vi "Drivetrain Loop.vi"() -> ()   [LabVIEW 2015]
uses:
  Common Code/Drivetrain Modes.ctl
  Common Code/Change Detect Boolean.vi
  Robot Global Data.vi
  <vilib>/Rock Robotics/WPI/Solenoid/Deprecated/WPI_SolenoidSetBool.vi
panel:
  out "Modes":T1=enum."Goal Vision Targeting"
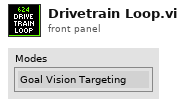
[diagram p1: front panel]
types:
  T1 = typedef "Drivetrain Modes.ctl" = enum16{"Gyro Steer", "Climb", "Manual", "Goal Vision Targeting", "PID Distance Drive", "Hybrid"}
  T2 = typedef "Drivetrain Commands.ctl" = cluster{"Y Power":dbl, "Turn Power":dbl, "Modes":T1, "Heading Target":dbl, "X Max Speed":dbl, "Y Max Speed":dbl, "X Min Speed":dbl, "Y Min Speed":dbl, "Y Target":dbl, "Max Accel":dbl, "Max Velocity":dbl, "Pivot Speed":dbl}
  T3 = typedef "WPI_DriverStationRobotMode2.ctl" = enum16{"Autonomous Disabled", "Autonomous Enabled", "Teleop Disabled", "Teleop Enabled", "Disconnected", "Finish", "Test Disabled", "Test Enabled", "Emergency Stopped"}
  T4 = typedef "Goal Vision Packet.ctl" = cluster{"Distance":dbl, "Center X":dbl, "Center Y":dbl, "Found Target?":bool, "Robot Center":dbl, "Angle":dbl}
  T5 = typedef "Dist Drive Status.ctl" = cluster{"Y In Range":bool, "X In Range":bool, "Gyro In Range":bool, "Y Dist":dbl, "X Dist":dbl, "Gyro":dbl}
  T6 = typedef "WPI_MotorControlDeviceRef.ctl" = cluster{"DeviceStatus":errorcluster, "Type":T7, "PWM":cluster{"PWM Channel":T8, "DeadBand":T9}, "CAN":cluster{"Device Number":u8, "Control Mode":T10, "Semaphore":T11, "Max Vout":dbl, "TalonSRX Control Mode":T12}, "Invert":bool}
  T7 = typedef "WPI_MotorControlType.ctl" = enum16{"PWM", "CAN", "CANTalonSRX"}
  T8 = typedef "FPGA_DIOPWMChannel.ctl" = enum8{"PWM 0", "PWM 1", "PWM 2", "PWM 3", "PWM 4", "PWM 5", "PWM 6", "PWM 7", "PWM 8", "PWM 9", "PWM MXP 0", "PWM MXP 1", "PWM MXP 2", "PWM MXP 3", "PWM MXP 4", "PWM MXP 5", "PWM MXP 6", "PWM MXP 7", "PWM MXP 8", "PWM MXP 9", "Invalid"}
  T9 = typedef "WPI_PWMDeadband.ctl" = cluster{"Name":string, "maxPositivePwm":i32, "minPositivePwm":i32, "centerPwm":i32, "maxNegativePwm":i32, "minNegativePwm":i32, "angularRange":u16}
  T10 = typedef "WPI_CANJaguar_ControlMode.ctl" = enum8{"Percent VBus", "Current", "Speed", "Position", "Voltage"}
  T11 = typedef "Semaphore RefNum" = refnum<k1>
  T12 = typedef "WPI_CANTalonSRX_APIControlMode.ctl" = enum8{"Percent VBus", "Speed", "Position", "Slave", "Unchanged / Invalid", "Voltage Compensation", "Current", "Motion Profile"}
  T13 = typedef "WPI_SolenoidDevRef.ctl" = cluster{"DevStatus":errorcluster, "Pneumatics Control Module":u8, "Forward Solenoid Channel":T14, "Reverse Solenoid Channel":T14}
  T14 = typedef "WPI_SolenoidChannel.ctl" = enum8{"Solenoid 0", "Solenoid 1", "Solenoid 2", "Solenoid 3", "Solenoid 4", "Solenoid 5", "Solenoid 6", "Solenoid 7", "Invalid"}
  T15 = typedef "Drivetrain Status Cluster.ctl" = cluster{"Modes":T1, "Y (Throttle)":dbl, "X (Steer)":dbl, "Gyro In Range?":bool, "Distance Drive Finished?":bool, "Stop Eject Lockout":bool, "Dist Drive Status":T5, "Y Target":dbl, "Heading Target":dbl, "Vision Target Aligned?":bool}
  T16 = typedef "Climb Status Cluster.ctl" = cluster{"Pull Power":dbl, "Unpin Power":dbl, "PTO Engaged?":bool, "Climb Mode":T17}
  T17 = typedef "Climb Mode.ctl" = enum16{"Auto", "Semi-Auto", "Manual"}
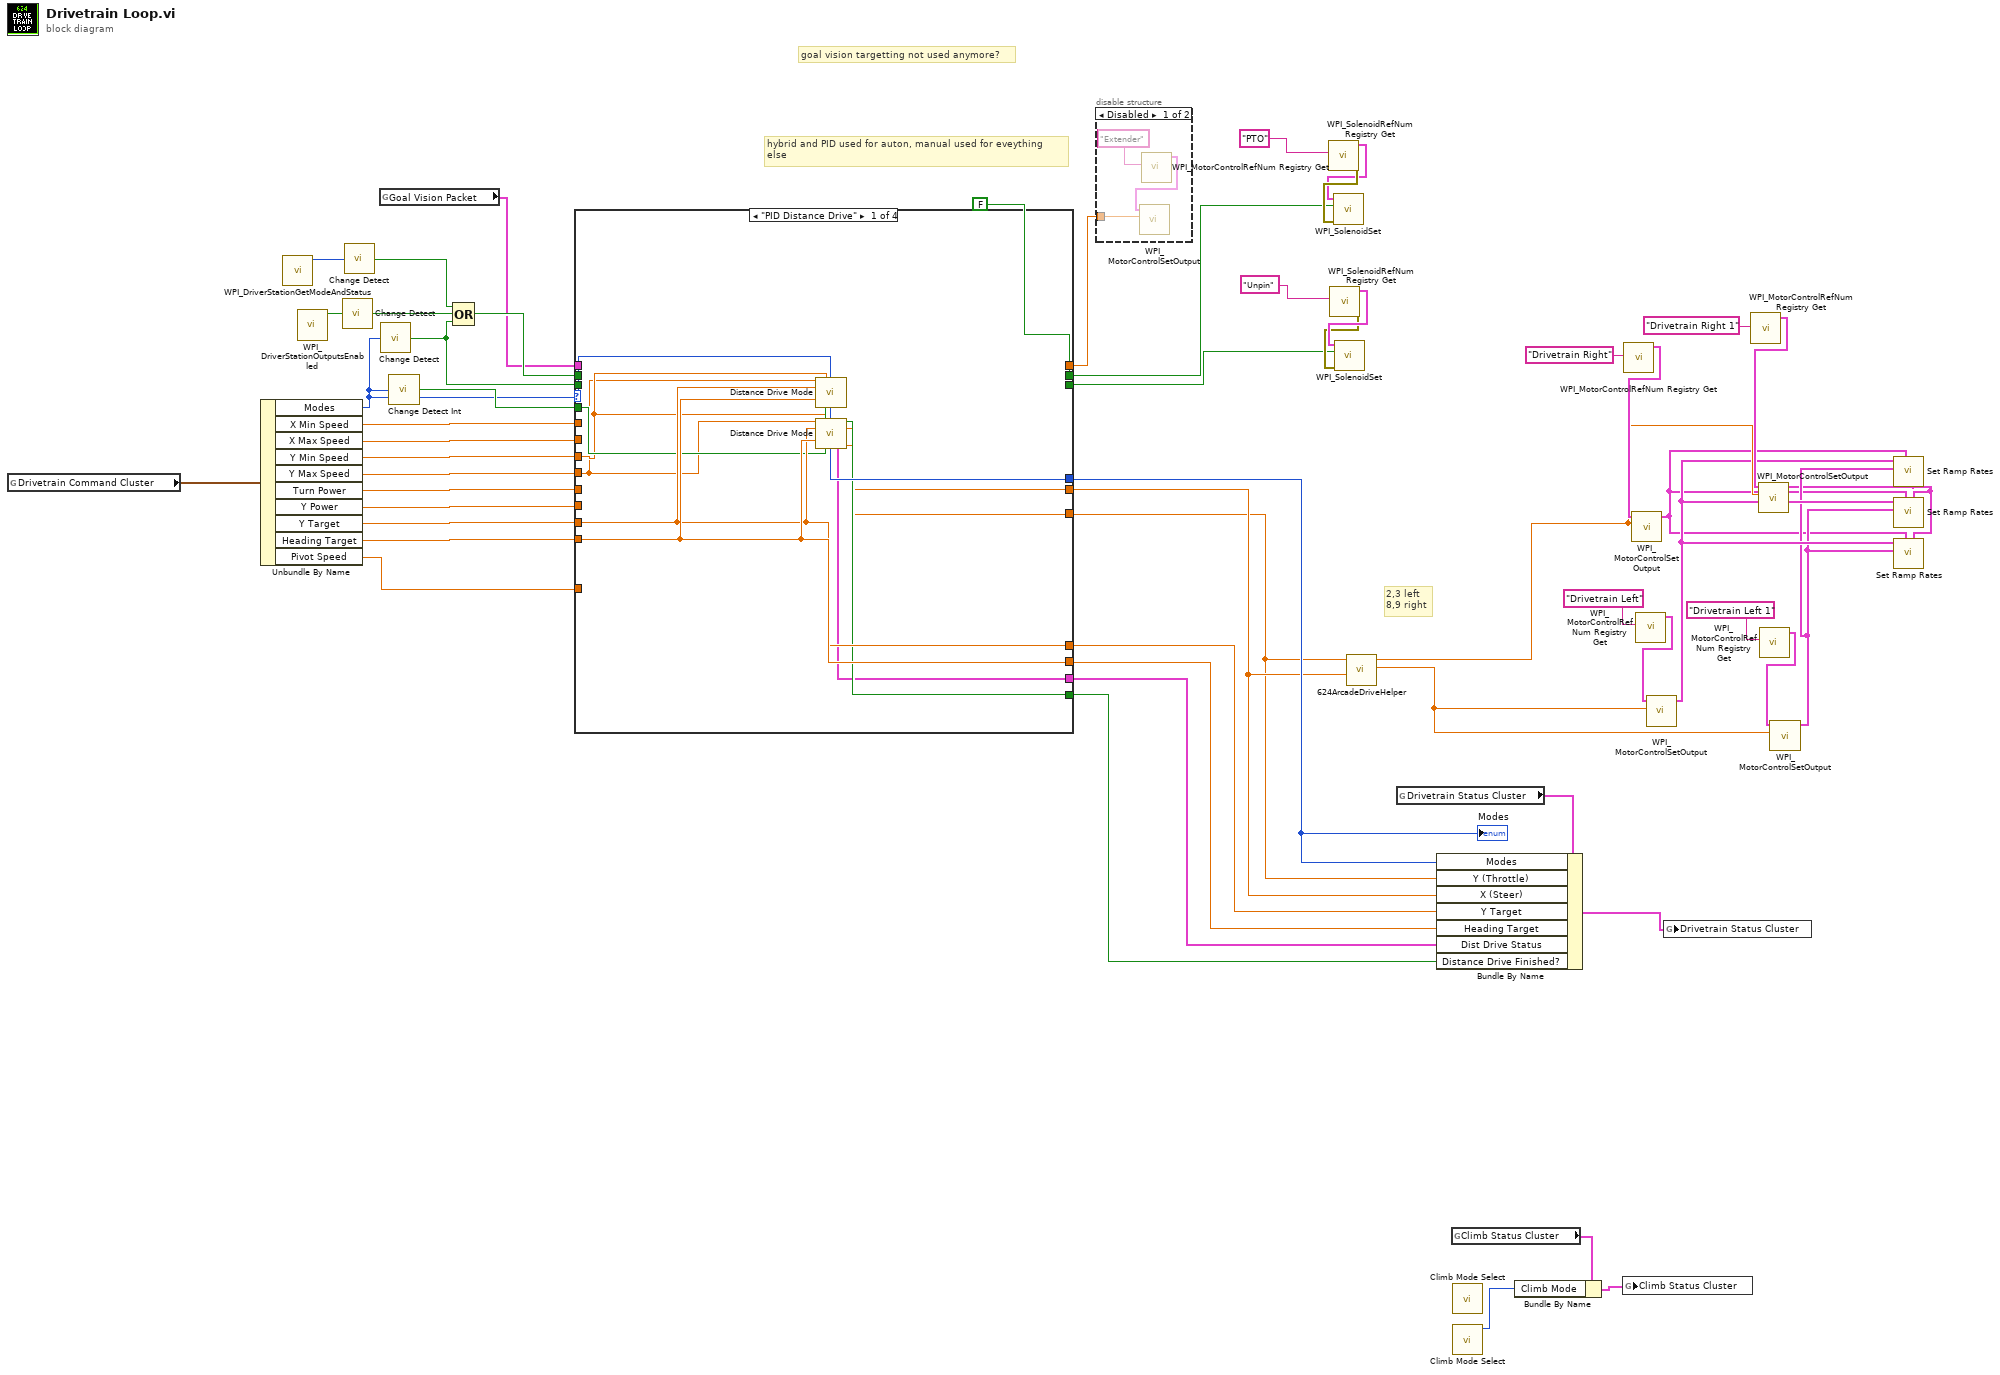
[diagram p0: block diagram]
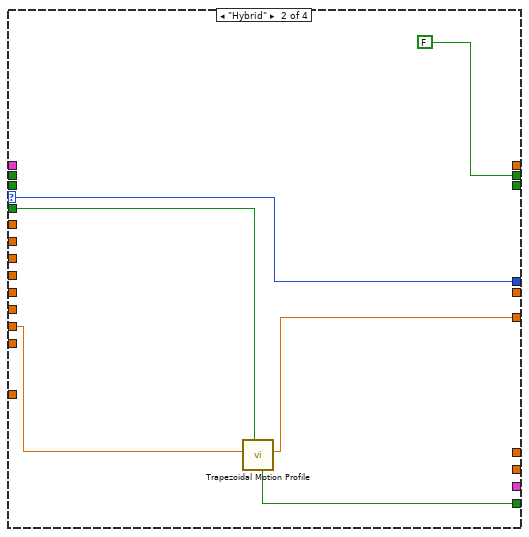
[diagram p3: hidden frame]
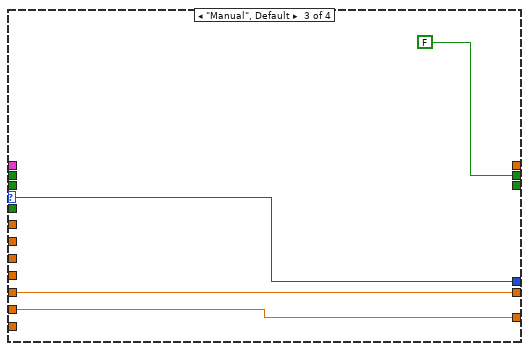
[diagram p4: hidden frame]
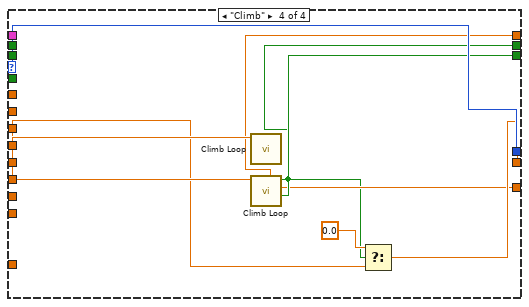
[diagram p5: hidden frame]
diagram:
  # "hybrid and PID used for auton, manual used for eveything \nelse"
  # "goal vision targetting not used anymore?"
  # "2,3 left\n8,9 right"
  n1 = global read "Robot Global Data.vi" "Drivetrain Command Cluster"() -> (w27:T2)
  n2 = Unbundle By Name(w27) -> ("Modes"=w26:T1, "X Min Speed"=w35:dbl, "X Max Speed"=w34:dbl, "Y Min Speed"=w33:dbl, "Y Max Speed"=w32:dbl, "Turn Power"=w31:dbl, "Y Power"=w30:dbl, "Y Target"=w29:dbl, "Heading Target"=w28:dbl, "Pivot Speed"=w2:dbl)
  n3 = call <vilib>:"WPI_DriverStationGetModeAndStatus.vi"() -> ("Robot Mode"=w15:T3)  [unwired: 10 in, 1 out]
  n4 = call <vilib>:"WPI_DriverStationOutputsEnabled.vi"() -> ("OutputsEnabled?"=w17:bool)  [unwired: 10 in, 1 out]
  n5 = call-poly "Change Detect.vi"("In"=w17) -> ("Changed?"=w16:bool)
  n6 = call-poly "Change Detect.vi"("In"=w15) -> ("Changed?"=w14:bool)
  n7 = global read "Robot Global Data.vi" "Goal Vision Packet"() -> (w4:T4)
  n8 = call-poly "Change Detect.vi"("In"=w26) -> ("Changed?"=w13:bool)
  n9 = call "Change Detect Int.vi"("In"=w26) -> ("Changed?"=w51:bool)
  n10 = Compound Arithmetic op=OR(w14, w16, w13) -> (w25:bool)
  n11 = case shown="\"PID Distance Drive\"" w26 {
    selector: w26 -> [w65 w66 w75 w84]
    tunnel: w35 -> [_ _ _ _]
    tunnel: w34 -> [_ _ _ _]
    tunnel: w33 -> [w60 _ _ _]
    tunnel: [w57 w71 w74 w78] -> w3
    tunnel: [w55 _ w72 w82] -> w24
    tunnel: [w65 w66 w75 w84] -> w54
    tunnel: w51 -> [w61 w69 _ _]
    tunnel: [w56 _ _ _] -> w46
    tunnel: [w58 w70 _ _] -> w47
    tunnel: [w63 _ _ _] -> w45
    tunnel: [w64 _ _ _] -> w44
    tunnel: w32 -> [w59 _ _ _]
    tunnel: w31 -> [_ _ w72 w80]
    tunnel: w30 -> [_ _ w74 w83]
    tunnel: w28 -> [w64 _ _ _]
    tunnel: w29 -> [w63 w68 _ _]
    tunnel: w4 -> [_ _ _ _]
    tunnel: [_ _ _ w76] -> w36
    tunnel: [FALSE ("PTO Engage") FALSE ("PTO Engage") FALSE ("PTO Engage") w77] -> w39
    tunnel: w2 -> [_ _ _ _]
    tunnel: w25 -> [_ _ _ _]
    tunnel: w13 -> [_ _ _ _]
    tunnel: [_ _ _ w79] -> w9
    frame "PID Distance Drive" {
      n12 = call "Distance Drive Mode.vi"("Y Output High"=w59, "Y Output Low"=w60, "Y target"=w63, "Heading target"=w64, "Reinitialize"=w61) -> ()  [unwired: 7 in, 4 out]
      n13 = call "Distance Drive Mode.vi"("Y Output High"=w59, "Y Output Low"=w60, "Y target"=w63, "Heading target"=w64, "Reinitialize"=w61) -> ("isFinished"=w58:bool, "Y out"=w57:dbl, "Dist Drive Status"=w56:T5, "X out"=w55:dbl)  [unwired: 7 in]
    }
    frame "Hybrid" {
      n14 = call "Trapezoidal Motion Profile.vi"("Reset?"=w69, "Distance"=w68) -> ("Throttle Out"=w71:sgl, "Finished?"=w70:bool)  [unwired: 8 in]
    }
    frame "Manual", Default {
    }
    frame "Climb" {
      n15 = call "Climb Loop.vi"("Y Power"=w83) -> ()  [unwired: 7 in, 4 out]
      n16 = call "Climb Loop.vi"("Y Power"=w83) -> ("Unpin?"=w79:bool, "Pull Power"=w78:dbl, "PTO Engaged?"=w77:bool, "Extend Power"=w76:dbl)  [unwired: 7 in]
      n17 = Select(t=0.0, s=w77, f=w80) -> (s? t:f=w82:dbl)
    }
  }
  "Modes" <- w54
  n18 = disable-structure shown="Disabled" {
    disable-tunnel: w36 -> [w87 _]
    frame Disabled {
      n19 = call <vilib>:"WPI_MotorControlRefNum Registry Get.vi"("refnum name"="Extender") -> ("MotorControlDevRef"=w86:T6)  [unwired: 9 in, 1 out]
      n20 = call <vilib>:"WPI_MotorControlSetOutput.vi"("Output"=w87, "MotorControlDevRef"=w86) -> ()  [unwired: 7 in, 3 out]
    }
    frame Enabled {
    }
  }
  n21 = call <vilib>:"WPI_SolenoidRefNum Registry Get.vi"("refnum name"="PTO") -> ("error out"=w42:errorcluster, "SolenoidDevRef"=w41:T13)  [unwired: 9 in]
  n22 = call <vilib>:"WPI_SolenoidRefNum Registry Get.vi"("refnum name"="Unpin") -> ("error out"=w10:errorcluster, "SolenoidDevRef"=w11:T13)  [unwired: 9 in]
  n23 = call-poly <vilib>:"WPI_SolenoidSet.vi"("error in (no error)"=w42, "Value"=w39, "SolenoidDevRef"=w41) -> ()  [unwired: 7 in, 2 out]
  n24 = call-poly <vilib>:"WPI_SolenoidSet.vi"("error in (no error)"=w10, "Value"=w9, "SolenoidDevRef"=w11) -> ()  [unwired: 7 in, 2 out]
  n25 = call "624ArcadeDriveHelper.vi"("Turn Power"=w24, "Y Power"=w3) -> ("Left"=w21:dbl, "Right"=w18:dbl)  [unwired: 8 in]
  n26 = global read "Robot Global Data.vi" "Drivetrain Status Cluster"() -> (w43:T15)
  n27 = Bundle By Name(cluster=w43, "Modes"=w54, "Y (Throttle)"=w3, "X (Steer)"=w24, "Y Target"=w45, "Heading Target"=w44, "Dist Drive Status"=w46, "Distance Drive Finished?"=w47) -> (w48:T15)
  n28 = global read "Robot Global Data.vi" "Climb Status Cluster"() -> (w37:T16)
  n29 = call "Climb Mode Select.vi"() -> ()  [unwired: 11 in, 1 out]
  n30 = call "Climb Mode Select.vi"() -> ("Mode"=w1:T17)  [unwired: 11 in]
  n31 = Bundle By Name(cluster=w37, "Climb Mode"=w1) -> (w38:T16)
  n32 = global write "Robot Global Data.vi" "Climb Status Cluster"(w38) -> ()
  n33 = call <vilib>:"WPI_MotorControlRefNum Registry Get.vi"("refnum name"="Drivetrain Right") -> ("MotorControlDevRef"=w50:T6)  [unwired: 9 in, 1 out]
  n34 = call <vilib>:"WPI_MotorControlSetOutput.vi"("Output"=w18, "MotorControlDevRef"=w50) -> ("MotorControlDevRef"=w6:T6)  [unwired: 7 in, 2 out]
  n35 = call <vilib>:"WPI_MotorControlRefNum Registry Get.vi"("refnum name"="Drivetrain Left") -> ("MotorControlDevRef"=w49:T6)  [unwired: 9 in, 1 out]
  n36 = call <vilib>:"WPI_MotorControlSetOutput.vi"("Output"=w21, "MotorControlDevRef"=w49) -> ("MotorControlDevRef"=w8:T6)  [unwired: 7 in, 2 out]
  n37 = global write "Robot Global Data.vi" "Drivetrain Status Cluster"(w48) -> ()
  n38 = call <vilib>:"WPI_MotorControlRefNum Registry Get.vi"("refnum name"="Drivetrain Right 1") -> ("MotorControlDevRef"=w20:T6)  [unwired: 9 in, 1 out]
  n39 = call <vilib>:"WPI_MotorControlSetOutput.vi"("Output"=w18, "MotorControlDevRef"=w20) -> ("MotorControlDevRef"=w5:T6)  [unwired: 7 in, 2 out]
  n40 = call <vilib>:"WPI_MotorControlRefNum Registry Get.vi"("refnum name"="Drivetrain Left 1") -> ("MotorControlDevRef"=w23:T6)  [unwired: 9 in, 1 out]
  n41 = call <vilib>:"WPI_MotorControlSetOutput.vi"("Output"=w21, "MotorControlDevRef"=w23) -> ("MotorControlDevRef"=w7:T6)  [unwired: 7 in, 2 out]
  n42 = call "Set Ramp Rates.vi"("DT Right 1"=w5, "DT Right"=w6, "DT Left 1"=w7, "DT Left"=w8) -> ()  [unwired: 8 in]
  n43 = call "Set Ramp Rates.vi"("DT Right 1"=w5, "DT Right"=w6, "DT Left 1"=w7, "DT Left"=w8) -> ()  [unwired: 8 in]
  n44 = call "Set Ramp Rates.vi"("DT Right 1"=w5, "DT Right"=w6, "DT Left 1"=w7, "DT Left"=w8) -> ()  [unwired: 8 in]
